vi "moveToPosition.vi"(0 "SingleAxisController in":refnum<class "_SingleAxisController.lvclass">, 2 "target(s) (in)":T1[](array[typedef]), 5 "error in (no error)":errorcluster) -> (14 "SingleAxisController out":refnum<class "_SingleAxisController.lvclass">, 17 "success?":bool, 18 "response":string, 19 "error out":errorcluster)   [LabVIEW 2020, in "classes.lvlib" / "_SingleAxisController.lvclass"]
doc: "Produced By:\n\n<B>Kod Integrations, LLC</B>\n4835 Marianne Drive\nMount Airy, MD 21771\nhttp://www.kodintegrations.com\nemail: info@kodintegrations.com\nphone: (240) 687-1288"
uses:
  _SingleAxisController.lvclass
  Controller/_Controller.lvclass
  C:/GEECS/Developers Version/source/Device Drivers/Newmark-NSC-A/Arcus Driver 3.0.0/ArcusUsbComm/classes/Controller/_Controller.lvclass
  C:/GEECS/Developers Version/source/Device Drivers/Newmark-NSC-A/Arcus Driver 3.0.0/ArcusUsbComm/classes/SingleAxisController/_SingleAxisController.lvclass
  common/controls/axis.ctl
  libraries/common.lvlib
  common/controls/movement_item.ctl
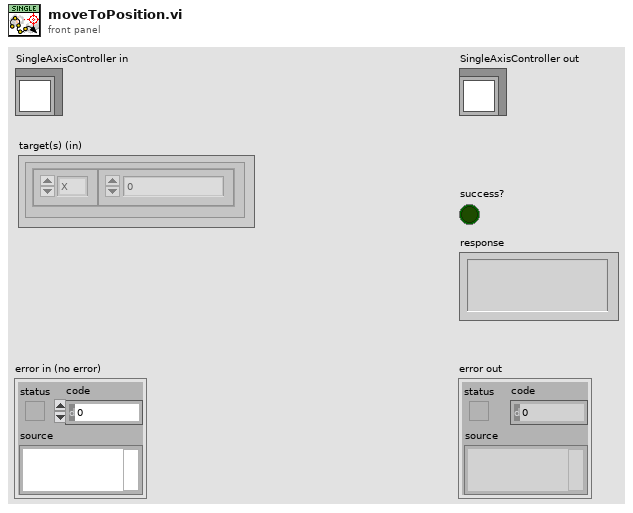
[diagram p1: front panel]
types:
  T1 = typedef "common.lvlib/movement_item.ctl" = cluster{"axis":T2, "target":i32}
  T2 = typedef "common.lvlib/axis.ctl" = enum16{"X", "Y", "Z", "U"}
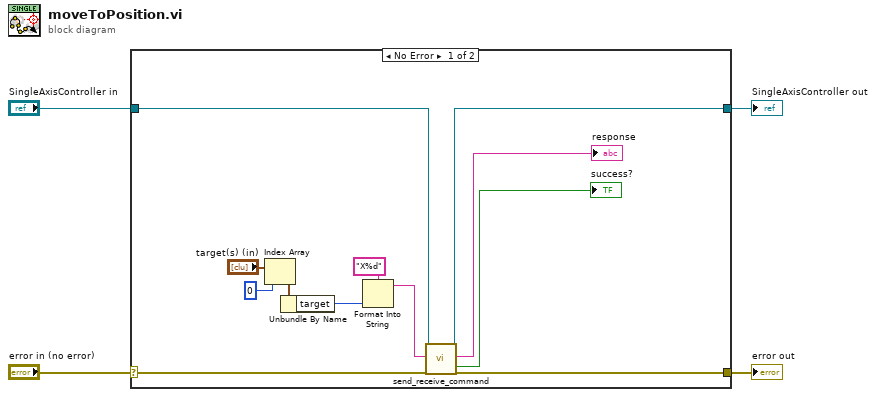
[diagram p0: block diagram]
diagram:
  n1 = case shown="No Error" "error in (no error)" {
    selector: "error in (no error)" -> [w12 w18]
    tunnel: [w11 w18] -> w3
    tunnel: [w9 w17] -> w1
    tunnel: "SingleAxisController in" -> [w10 w17]
    frame No Error {
      n2 = Index Array(array="target(s) (in)", index=0) -> (element=w6:T1)
      n3 = Unbundle By Name(w6) -> ("target"=w5:i32)
      n4 = Format Into String(format string="X%d", w5) -> (resulting string=w15:string)  [unwired: 2 in, 1 out]
      n5 = call "send_receive_command.vi"("reference (in)"=w10, "ASCII Command (in)"=w15, "error in (no error)"=w12) -> ("reference (out)"=w9:refnum<class "_SingleAxisController.lvclass">, "response (out)"=→"response":string, "success?"=→"success?":bool, "error out"=w11:errorcluster)  [unwired: 12 in, 1 out]
    }
    frame Error {
    }
  }
  "error out" <- w3
  "SingleAxisController out" <- w1
